vi "9235_9236_9237 8Ch Analog Input.vi"(1 "9235/9236/9237 I/O":T1={"9235/9236/9237 AI0"="NI 9235/AI0", "9235/9236/9237 AI1"="NI 9235/AI1", "9235/9236/9237 AI2"="NI 9235/AI2", "9235/9236/9237 AI3"="NI 9235/AI3", "9235/9236/9237 AI4"="NI 9235/AI4", "9235/9236/9237 AI5"="NI 9235/AI5", "9235/9236/9237 AI6"="NI 9235/AI6", "9235/9236/9237 AI7"="NI 9235/AI7"}) -> (0 "Packets":u64[](array[numeric]))   [LabVIEW 2010]
uses:
  <vilib>/eio/EIONode/EIONode.xnode
  <vilib>/rvi/eio/nirviEIOImplementation/nirviEIOImplementation.xnode
  <vilib>/rvi/eio/common/nirviEmuClasses.ctl
  <vilib>/rvi/eio/common/nirviEmuTemplateMethod_noerrors.vi
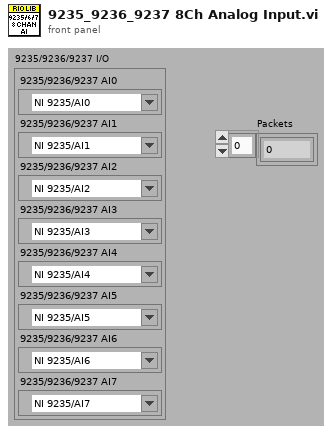
[diagram p1: front panel]
types:
  T1 = cluster{"9235/9236/9237 AI0":refnum<k21>, "9235/9236/9237 AI1":refnum<k21>, "9235/9236/9237 AI2":refnum<k21>, "9235/9236/9237 AI3":refnum<k21>, "9235/9236/9237 AI4":refnum<k21>, "9235/9236/9237 AI5":refnum<k21>, "9235/9236/9237 AI6":refnum<k21>, "9235/9236/9237 AI7":refnum<k21>}
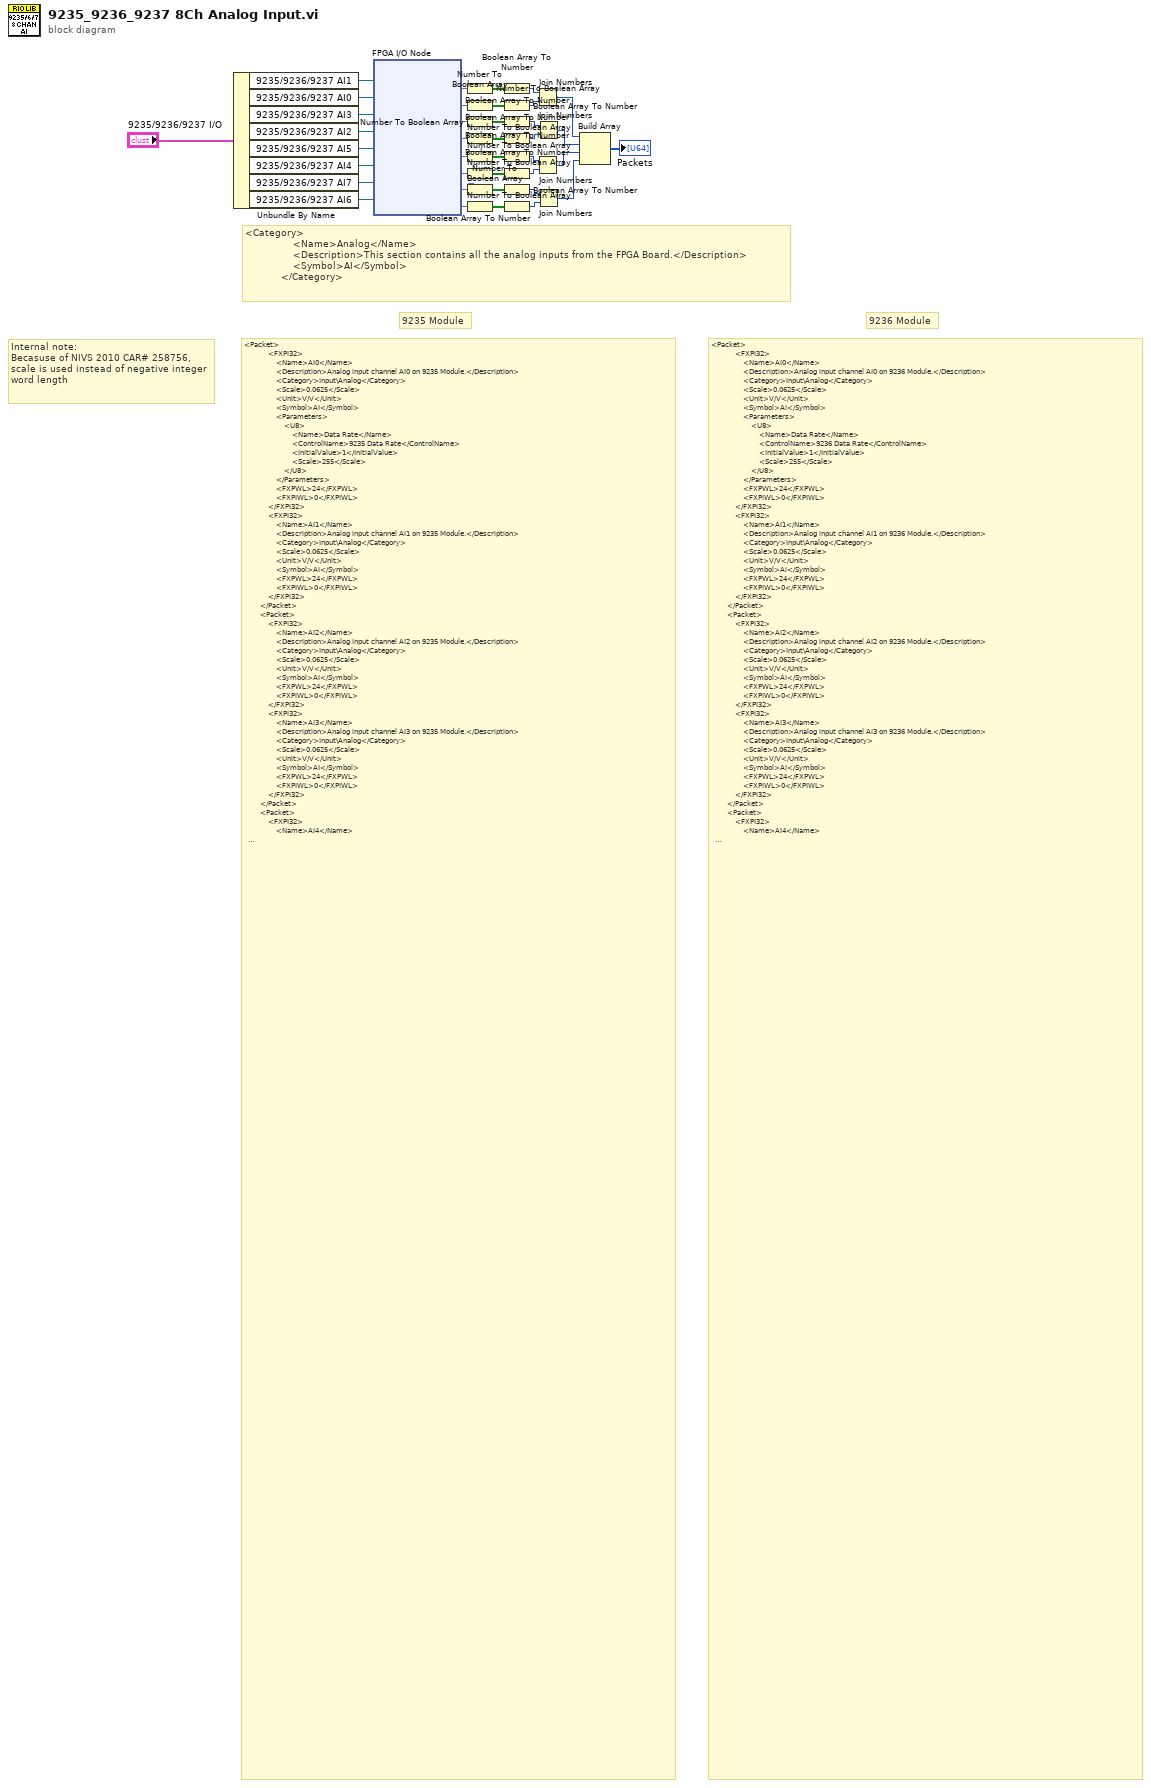
[diagram p0: block diagram]
diagram:
  # "9236 Module"
  # "<Packet>\n            <FXPI32>\n                <Name>AI0</Name>\n                <Description>Analog input channel AI0 on 9236 Module.</Description>\n                <Category>Input\\Analog</Category>\n                <Scale>0.0625</Scale>\n                <Unit>V/V</Unit>\n                <Symbol>AI</Symbol>\n                <Parameters>\n                    <U8>\n                        <Name>Data Rate</Name>\n                        <ControlName>9236 Data Rate</ControlName>\n                        <InitialValue>1</InitialValue>\n                        <Scale>255</Scale>\n                    </U8>\n                </Parameters>\n                <FXPWL>24</FXPWL>\n                <FXPIWL>0</FXPIWL>\n            </FXPI32>\n            <FXPI32>\n                <Name>AI1</Name>\n                <Description>Analog input channel AI1 on 9236 Module.</Description>\n                <Category>Input\\Analog</Category>\n                <Scale>0.0625</Scale>\n                <Unit>V/V</Unit>\n                <Symbol>AI</Symbol>\n                <FXPWL>24</FXPWL>\n                <FXPIWL>0</FXPIWL>\n            </FXPI32>\n        </Packet>\n        <Packet>\n            <FXPI32>\n                <Name>AI2</Name>\n                <Description>Analog input channel AI2 on 9236 Module.</Description>\n                <Category>Input\\Analog</Category>\n                <Scale>0.0625</Scale>\n                <Unit>V/V</Unit>\n                <Symbol>AI</Symbol>\n                <FXPWL>24</FXPWL>\n                <FXPIWL>0</FXPIWL>\n            </FXPI32>\n            <FXPI32>\n                <Name>AI3</Name>\n                <Description>Analog input channel AI3 on 9236 Module.</Description>\n                <Category>Input\\Analog</Category>\n                <Scale>0.0625</Scale>\n                <Unit>V/V</Unit>\n                <Symbol>AI</Symbol>\n                <FXPWL>24</FXPWL>\n                <FXPIWL>0</FXPIWL>\n            </FXPI32>\n        </Packet>\n        <Packet>\n            <FXPI32>\n                <Name>AI4</Name>\n                <Description>Analog input channel AI4 on 9236 Module.</Description>\n                <Category>Input\\Analog</Category>\n                <Scale>0.0625</Scale>\n                <Unit>V/V</Unit>\n                <Symbol>AI</Symbol>\n                <FXPWL>24</FXPWL>\n                <FXPIWL>0</FXPIWL>\n            </FXPI32>\n            <FXPI32>\n                <Name>AI5</Name>\n                <Description>Analog input channel AI5 on 9236 Module.</Description>\n                <Category>Input\\Analog</Category>\n                <Scale>0.0625</Scale>\n                <Unit>V/V</Unit>\n                <Symbol>AI</Symbol>\n                <FXPWL>24</FXPWL>\n                <FXPIWL>0</FXPIWL>\n            </FXPI32>\n        </Packet>\n        <Packet>\n            <FXPI32>\n                <Name>AI6</Name>\n                <Description>Analog input channel AI6 on 9236 Module.</Description>\n                <Category>Input\\Analog</Category>\n                <Scale>0.0625</Scale>\n                <Unit>V/V</Unit>\n                <Symbol>AI</Symbol>\n                <FXPWL>24</FXPWL>\n                <FXPIWL>0</FXPIWL>\n            </FXPI32>\n            <FXPI32>\n                <Name>AI7</Name>\n                <Description>Analog input channel AI7 on 9236 Module.</Description>\n                <Category>Input\\Analog</Category>\n                <Scale>0.0625</Scale>\n                <Unit>V/V</Unit>\n                <Symbol>AI</Symbol>\n                <FXPWL>24</FXPWL>\n                <FXPIWL>0</FXPIWL>\n            </FXPI32>\n        </Packet>"
  # "9235 Module"
  # "Internal note:\nBecasuse of NIVS 2010 CAR# 258756, scale is used instead of negative integer word length"
  # "<Category>\n                <Name>Analog</Name>\n                <Description>This section contains all the analog inputs from the FPGA Board.</Description>\n                <Symbol>AI</Symbol>\n            </Category>"
  # "<Packet>\n            <FXPI32>\n                <Name>AI0</Name>\n                <Description>Analog input channel AI0 on 9235 Module.</Description>\n                <Category>Input\\Analog</Category>\n                <Scale>0.0625</Scale>\n                <Unit>V/V</Unit>\n                <Symbol>AI</Symbol>\n                <Parameters>\n                    <U8>\n                        <Name>Data Rate</Name>\n                        <ControlName>9235 Data Rate</ControlName>\n                        <InitialValue>1</InitialValue>\n                        <Scale>255</Scale>\n                    </U8>\n                </Parameters>\n                <FXPWL>24</FXPWL>\n                <FXPIWL>0</FXPIWL>\n            </FXPI32>\n            <FXPI32>\n                <Name>AI1</Name>\n                <Description>Analog input channel AI1 on 9235 Module.</Description>\n                <Category>Input\\Analog</Category>\n                <Scale>0.0625</Scale>\n                <Unit>V/V</Unit>\n                <Symbol>AI</Symbol>\n                <FXPWL>24</FXPWL>\n                <FXPIWL>0</FXPIWL>\n            </FXPI32>\n        </Packet>\n        <Packet>\n            <FXPI32>\n                <Name>AI2</Name>\n                <Description>Analog input channel AI2 on 9235 Module.</Description>\n                <Category>Input\\Analog</Category>\n                <Scale>0.0625</Scale>\n                <Unit>V/V</Unit>\n                <Symbol>AI</Symbol>\n                <FXPWL>24</FXPWL>\n                <FXPIWL>0</FXPIWL>\n            </FXPI32>\n            <FXPI32>\n                <Name>AI3</Name>\n                <Description>Analog input channel AI3 on 9235 Module.</Description>\n                <Category>Input\\Analog</Category>\n                <Scale>0.0625</Scale>\n                <Unit>V/V</Unit>\n                <Symbol>AI</Symbol>\n                <FXPWL>24</FXPWL>\n                <FXPIWL>0</FXPIWL>\n            </FXPI32>\n        </Packet>\n        <Packet>\n            <FXPI32>\n                <Name>AI4</Name>\n                <Description>Analog input channel AI4 on 9235 Module.</Description>\n                <Category>Input\\Analog</Category>\n                <Scale>0.0625</Scale>\n                <Unit>V/V</Unit>\n                <Symbol>AI</Symbol>\n                <FXPWL>24</FXPWL>\n                <FXPIWL>0</FXPIWL>\n            </FXPI32>\n            <FXPI32>\n                <Name>AI5</Name>\n                <Description>Analog input channel AI5 on 9235 Module.</Description>\n                <Category>Input\\Analog</Category>\n                <Scale>0.0625</Scale>\n                <Unit>V/V</Unit>\n                <Symbol>AI</Symbol>\n                <FXPWL>24</FXPWL>\n                <FXPIWL>0</FXPIWL>\n            </FXPI32>\n        </Packet>\n        <Packet>\n            <FXPI32>\n                <Name>AI6</Name>\n                <Description>Analog input channel AI6 on 9235 Module.</Description>\n                <Category>Input\\Analog</Category>\n                <Scale>0.0625</Scale>\n                <Unit>V/V</Unit>\n                <Symbol>AI</Symbol>\n                <FXPWL>24</FXPWL>\n                <FXPIWL>0</FXPIWL>\n            </FXPI32>\n            <FXPI32>\n                <Name>AI7</Name>\n                <Description>Analog input channel AI7 on 9235 Module.</Description>\n                <Category>Input\\Analog</Category>\n                <Scale>0.0625</Scale>\n                <Unit>V/V</Unit>\n                <Symbol>AI</Symbol>\n                <FXPWL>24</FXPWL>\n                <FXPIWL>0</FXPIWL>\n            </FXPI32>\n        </Packet>"
  n1 = Unbundle By Name("9235/9236/9237 I/O") -> ("9235/9236/9237 AI1"=w23:refnum<k21>, "9235/9236/9237 AI0"=w26:refnum<k21>, "9235/9236/9237 AI3"=w24:refnum<k21>, "9235/9236/9237 AI2"=w27:refnum<k21>, "9235/9236/9237 AI5"=w15:refnum<k21>, "9235/9236/9237 AI4"=w16:refnum<k21>, "9235/9236/9237 AI7"=w17:refnum<k21>, "9235/9236/9237 AI6"=w18:refnum<k21>)
  n2 = xnode "FPGA I/O Node"("FPGA I/O In"=w23, "FPGA I/O In"=w26, "FPGA I/O In"=w24, "FPGA I/O In"=w27, "FPGA I/O In"=w15, "FPGA I/O In"=w16, "FPGA I/O In"=w17, "FPGA I/O In"=w18) -> ("I/O Item"=w32:fxp<+/-,24,-4>, "I/O Item"=w34:fxp<+/-,24,-4>, "I/O Item"=w25:fxp<+/-,24,-4>, "I/O Item"=w33:fxp<+/-,24,-4>, "I/O Item"=w3:fxp<+/-,24,-4>, "I/O Item"=w4:fxp<+/-,24,-4>, "I/O Item"=w5:fxp<+/-,24,-4>, "I/O Item"=w6:fxp<+/-,24,-4>)  [unwired: 8 out]
  n3 = Number To Boolean Array(number=w32) -> (Boolean array=w28:bool[])
  n4 = Number To Boolean Array(number=w34) -> (Boolean array=w29:bool[])
  n5 = Number To Boolean Array(number=w25) -> (Boolean array=w31:bool[])
  n6 = Number To Boolean Array(number=w33) -> (Boolean array=w30:bool[])
  n7 = Number To Boolean Array(number=w3) -> (Boolean array=w14:bool[])
  n8 = Number To Boolean Array(number=w4) -> (Boolean array=w13:bool[])
  n9 = Number To Boolean Array(number=w5) -> (Boolean array=w11:bool[])
  n10 = Number To Boolean Array(number=w6) -> (Boolean array=w12:bool[])
  n11 = Boolean Array To Number(Boolean array=w28) -> (number=w35:u32)
  n12 = Boolean Array To Number(Boolean array=w29) -> (number=w36:u32)
  n13 = Boolean Array To Number(Boolean array=w31) -> (number=w37:u32)
  n14 = Boolean Array To Number(Boolean array=w30) -> (number=w38:u32)
  n15 = Boolean Array To Number(Boolean array=w14) -> (number=w10:u32)
  n16 = Boolean Array To Number(Boolean array=w13) -> (number=w9:u32)
  n17 = Boolean Array To Number(Boolean array=w11) -> (number=w8:u32)
  n18 = Boolean Array To Number(Boolean array=w12) -> (number=w7:u32)
  n19 = Join Numbers(hi=w35, lo=w36) -> ((hi.lo)=w21:u64)
  n20 = Join Numbers(hi=w10, lo=w9) -> ((hi.lo)=w2:u64)
  n21 = Join Numbers(hi=w37, lo=w38) -> ((hi.lo)=w22:u64)
  n22 = Join Numbers(hi=w8, lo=w7) -> ((hi.lo)=w1:u64)
  n23 = Build Array(w21, w22, w2, w1) -> (→"Packets":u64[])
